vi "readU32.vi"(8 "error in (no error)":errorcluster, 9 "Timeout":i32, 10 "NumberOfElements":u32, 11 "MyHealthAndStatusReadFIFO in":refnum<class "ModbusPort1ReadFIFO.lvclass">) -> (0 "error out":errorcluster, 1 "ElementsRemaining":u32, 2 "Data":u32[](array[numeric]), 3 "MyHealthAndStatusReadFIFO out":refnum<class "ModbusPort1ReadFIFO.lvclass">)   [LabVIEW 2015]
uses:
  <vilib>/rvi/interface/nirviMethod/nirviMethod.xnode
  <vilib>/FPGAPlugInAG/Dynamic/niLvFpga_ReadFifo_Dynamic.vi
  <vilib>/rvi/errors/niLvFpgaMergeErrorWithErrorCode.vi
  ModbusPort1ReadFIFO.lvclass
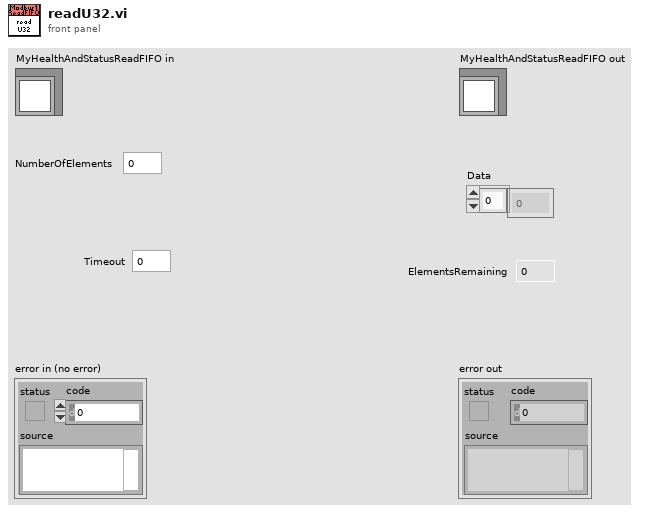
[diagram p1: front panel]
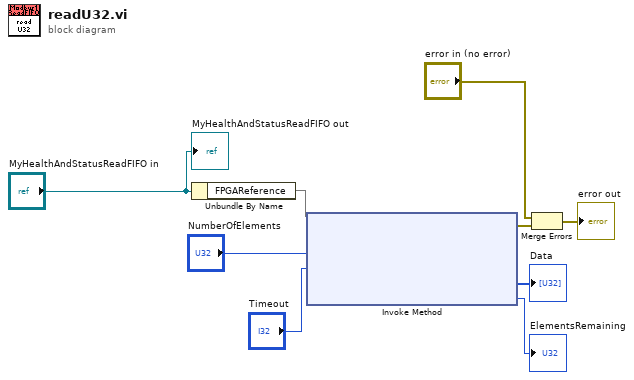
[diagram p0: block diagram]
diagram:
  n1 = Unbundle By Name("MyHealthAndStatusReadFIFO in") -> ("FPGAReference"=w9)
  n2 = xnode "Invoke Method"("FPGA VI Reference In"=w9, "Number of Elements"="NumberOfElements", "Timeout (ms)"="Timeout") -> ("error out"=w2:errorcluster, "Data"=→"Data":u32[], "Elements Remaining"=→"ElementsRemaining":u32)  [unwired: 1 in, 1 out]
  n3 = Merge Errors("error in (no error)", w2) -> (→"error out":errorcluster)
  "MyHealthAndStatusReadFIFO out" <- "MyHealthAndStatusReadFIFO in"
